vi "DHE_setup_image.vi"(6 "raw bpp":i32=16, 8 "error in (no error)":errorcluster, 10 "usc present":bool, 11 "Database RefNum in":T1) -> (0 "error out":errorcluster)   [LabVIEW 2016]
uses:
  DBSHAND/private/vis/DatabaseHand_RefNum.ctl
  DBSHAND/private/vis/DatabaseHand_Element_Get(string).vi
  DBSHAND/private/vis/DatabaseHand_Element_Get(I32).vi
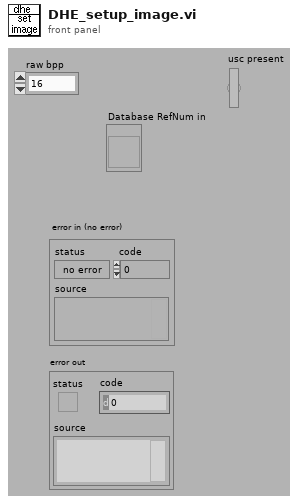
[diagram p1: front panel]
types:
  T1 = typedef "DatabaseHand_RefNum.ctl" = refnum<vi>
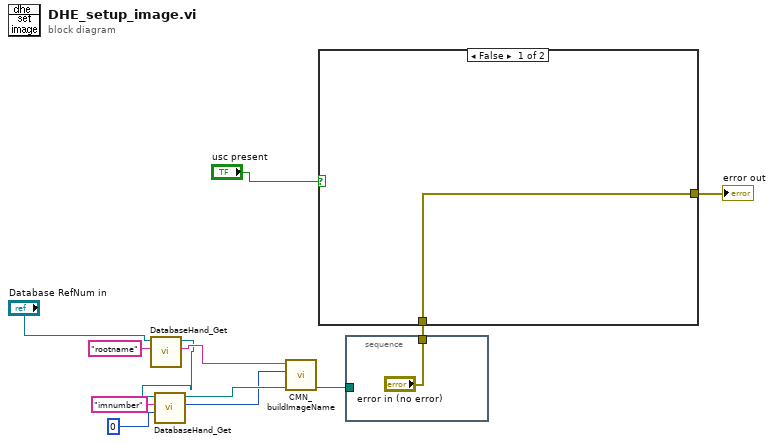
[diagram p0: block diagram]
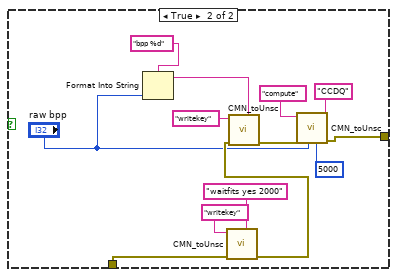
[diagram p2: hidden frame]
diagram:
  n1 = call-poly "DatabaseHand_Get.vi"("name"="rootname", "Database RefNum in"="Database RefNum in") -> ("value"=w10:string, "Database RefNum out"=w9:T1)  [unwired: 3 in, 5 out]
  n2 = call-poly "DatabaseHand_Get.vi"("default value"=0, "name"="imnumber", "Database RefNum in"=w9) -> ("value"=w6:i32, "Database RefNum out"=w11:T1)  [unwired: 2 in, 5 out]
  n3 = call "CMN_buildImageName.vi"("Database RefNum out"=w11, "imageNumber"=w6, "root name"=w10) -> ("Path out"=w2:path)  [unwired: 1 in, 5 out]
  n4 = stacked-sequence {
    tunnel: ["error in (no error)"] -> w3
    tunnel: w2 -> [_]
    frame #0 {
    }
  }
  n5 = case shown="False" "usc present" {
    tunnel: [w14 w16] -> w4
    tunnel: w3 -> [w14 w15]
    frame False {
    }
    frame True {
      n6 = Format Into String(format string="bpp %d" ("key"), "raw bpp") -> (resulting string=w18:string)  [unwired: 2 in, 1 out]
      n7 = call "CMN_toUnsc.vi"("key"="waitfits yes 2000", "error in (no error)"=w15, "command"="writekey") -> ("error out"=w21:errorcluster)  [unwired: 6 in, 2 out]
      n8 = call "CMN_toUnsc.vi"("key"=w18, "error in (no error)"=w21, "command"="writekey") -> ("error out"=w26:errorcluster)  [unwired: 6 in, 2 out]
      n9 = call "CMN_toUnsc.vi"("responseQ"="CCDQ", "ms timeout (-1)"=5000, "bpp"="raw bpp", "error in (no error)"=w26, "command"="compute") -> ("error out"=w16:errorcluster)  [unwired: 4 in, 2 out]
    }
  }
  "error out" <- w4
